vi "Test Convert.vi"(11 "Error in":errorcluster) -> (15 "Error out":errorcluster)   [LabVIEW 2020, in "CelsiusToFarenheitTests.lvlib"]
doc: "This VI is to validate Celsius to farenheit"
uses:
  CelsiusToFarenheitTests.lvlib
  <vilib>/addons/_JKI Toolkits/Caraya/classes/Test Suite/Define Test Suite (JUnit Report).vi
  <vilib>/SLL Drona/APIs/Stimulus/ControlValue/ValueSignalByPathString.vi
  <vilib>/SLL Drona/APIs/Assert/AssertControlValue/AlmostEqual.vi
  <vilib>/SLL Drona/APIs/Stimulus/VI/CloseVI.vi
  <vilib>/Utility/error.llb/Error Cluster From Error Code.vi
  <vilib>/ErrorRing/Error Ring.xnode
  <vilib>/addons/_JKI Toolkits/Caraya/classes/Test Suite/Test Suite.lvclass
  <vilib>/SLL Drona/Drona.lvlib
  <vilib>/addons/_JKI Toolkits/Caraya/classes/Test/Test.lvclass
  <vilib>/Wiresmith Technology/G CLI/CLI Class/CLI.lvclass
  <vilib>/SLL Drona/APIs/Assert/AssertControlValue/AssertControlValue.lvlib
  <vilib>/SLL Drona/APIs/Stimulus/ControlValue/ControlValue.lvlib
  <vilib>/SLL Drona/APIs/Stimulus/VI/VI.lvlib
panel:
  # "CELSIUS TO FARENHEIT TEST"
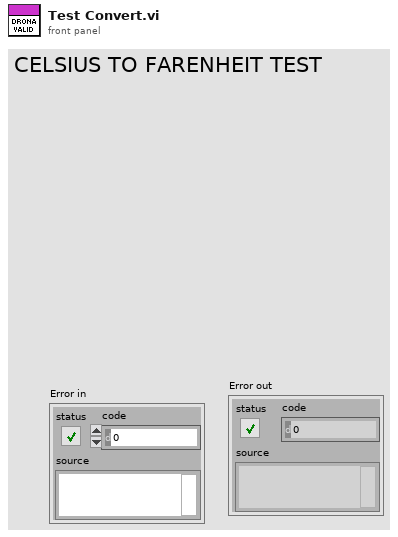
[diagram p1: front panel]
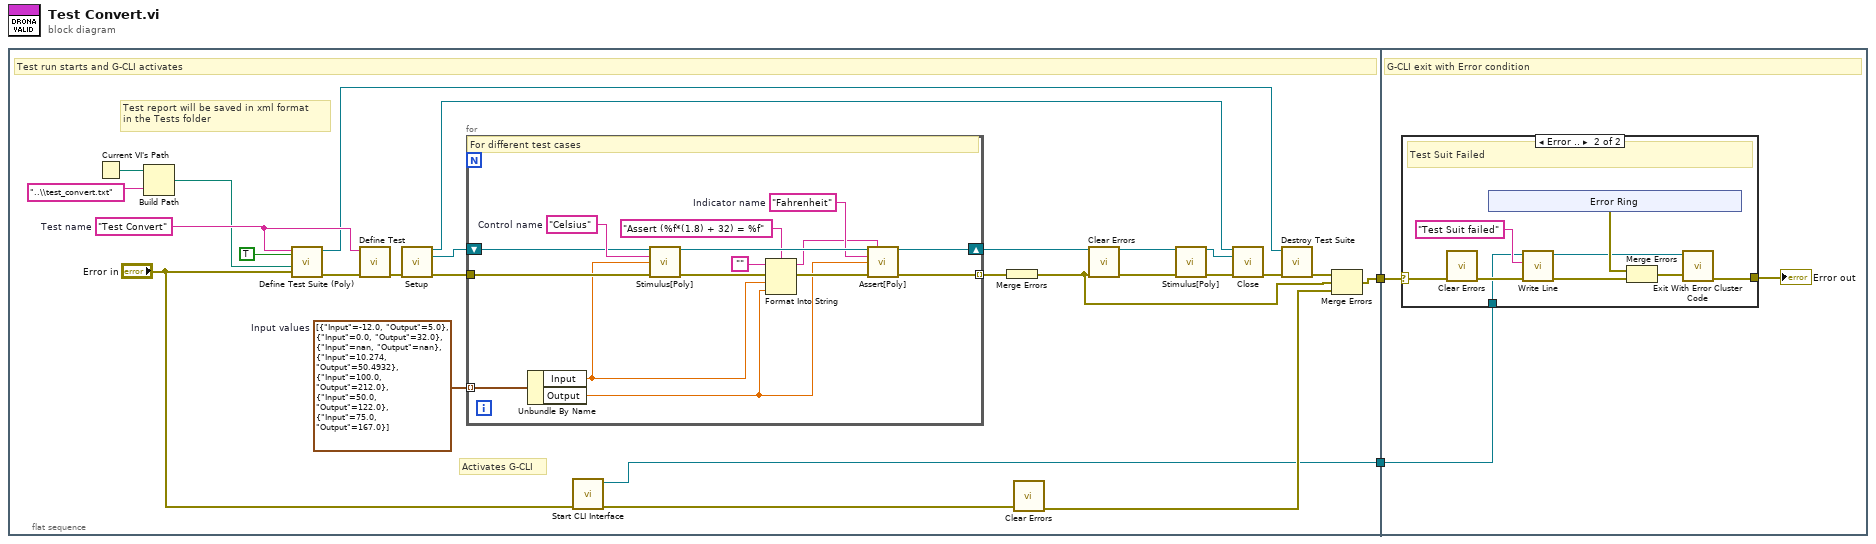
[diagram p0: block diagram]
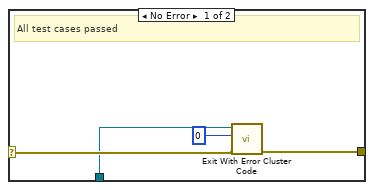
[diagram p2: hidden frame]
diagram:
  n1 = flat-sequence {
    tunnel: [w17] -> w2
    tunnel: [w15] -> w1
    tunnel: w2 -> [w45]
    tunnel: w1 -> [w43]
    frame #0 {
      w14 = "Test Convert"  # Test name
      w25 = cluster{"Input":dbl, "Output":dbl}[] [{"Input"=-12.0, "Output"=5.0}, {"Input"=0.0, "Output"=32.0}, {"Input"=nan, "Output"=nan}, {"Input"=10.274, "Output"=50.4932}, {"Input"=100.0, "Output"=212.0}, {"Input"=50.0, "Output"=122.0}, {"Input"=75.0, "Output"=167.0}]  # Input values
      # "Test report will be saved in xml format\nin the Tests folder"
      # "Activates G-CLI"
      # "Test run starts and G-CLI activates"
      n2 = Current VI's Path() -> (path=w10:path)
      n3 = Build Path(base path=w10, name or relative path="..\\test_convert.txt") -> (appended path=w8:path)
      n4 = call-poly <vilib>:"Define Test Suite (Poly).vi"("error in (no error)"="Error in", "Report Path"=w8, "Interactive"=TRUE, "Label (VI Title)"=w14) -> ("error out"=w13:errorcluster, "Test Suite"=w5:refnum<class "Test Suite.lvclass">)  [unwired: 6 in]
      n5 = call <vilib>:"Define Test.vi"("error in (no error)"=w13, "Label (VI Title)"=w14) -> ("error out"=w27:errorcluster)  [unwired: 9 in]
      n6 = call <vilib>:"Setup.vi"("error in"=w27) -> ("Application Ref"=w23:refnum<vi>, "VI Reference Out"=w24:refnum<vi>, "error out"=w26:errorcluster)  [unwired: 12 in]
      n7 = for {
        tunnel: w25 -> [w41] mode=indexing
        shift-right: [w31] -> w22
        shift-left: w24 -> [w39]
        tunnel: w26 -> [w42]
        tunnel: [w29] -> w19 mode=indexing
        w32 = "Fahrenheit"  # Indicator name
        w40 = "Celsius"  # Control name
        # "For different test cases"
        n8 = Unbundle By Name(w41) -> ("Input"=w28:dbl, "Output"=w33:dbl)
        n9 = call-poly <vilib>:"Stimulus[Poly].vi"("VI Reference In"=w39, "Control Path"=w40, "Value (Signaling)"=w28, "error in"=w42) -> ("VI Reference Out"=w35:refnum<vi>, "error out"=w37:errorcluster)  [unwired: 10 in]
        n10 = Format Into String(format string="Assert (%f*(1.8) + 32) = %f", initial string="", error in=w37, w28, w33) -> (resulting string=w30:string, error out=w36:errorcluster)
        n11 = call-poly <vilib>:"Assert[Poly].vi"("VI Reference In"=w35, "Test Label"=w30, "Control Path"=w32, "Control Value"=w33, "Error In"=w36) -> ("VI Reference Out"=w31:refnum<vi>, "Error Out"=w29:errorcluster)  [unwired: 9 in]
      }
      n12 = call <vilib>:"Start CLI Interface.vi"("error in (no error)"="Error in") -> ("error out"=w16:errorcluster, "CLI out"=w15:refnum<class "CLI.lvclass">)  [unwired: 7 in, 2 out]
      n13 = Merge Errors(w19) -> (w3:errorcluster)
      n14 = call <vilib>:"Clear Errors.vi"("error in (no error)"=w16) -> ("error out"=w18:errorcluster)  [unwired: 5 in, 1 out]
      n15 = call <vilib>:"Clear Errors.vi"("error in (no error)"=w3) -> ("error out"=w4:errorcluster)  [unwired: 5 in, 1 out]
      n16 = call-poly <vilib>:"Stimulus[Poly].vi"("VI Reference In"=w22, "error in"=w4) -> ("VI Reference Out"=w21:refnum<vi>, "error out"=w20:errorcluster)  [unwired: 12 in]
      n17 = call <vilib>:"Close.vi"("Application Ref"=w23, "VI Reference"=w21, "error in"=w20) -> ("error out"=w7:errorcluster)  [unwired: 12 in]
      n18 = call-dynamic "Destroy Test Suite.vi"("error in (no error)"=w7, "Test Suite in"=w5) -> ("error out"=w6:errorcluster)  [unwired: 8 in, 1 out]
      n19 = Merge Errors(w6, w3, w18) -> (w17:errorcluster)
    }
    frame #1 {
      # "G-CLI exit with Error condition"
      n20 = case shown="Error .." w45 {
        selector: w45 -> [w49 w56]
        tunnel: [w48 w58] -> w44
        tunnel: w43 -> [w46 w51]
        frame No Error {
          # "All test cases passed"
          n21 = call <vilib>:"Exit With Error Cluster Code.vi"("error in (no error)"=w49, "No Error Code (0)"=0, "CLI in"=w46) -> ("error out"=w48:errorcluster)  [unwired: 8 in]
        }
        frame Error {
          # "Test Suit Failed"
          n22 = call <vilib>:"Clear Errors.vi"("error in (no error)"=w56) -> ("error out"=w55:errorcluster)  [unwired: 5 in, 1 out]
          n23 = xnode "Error Ring"() -> ("error out"=w53:errorcluster)
          n24 = call <vilib>:"Write Line.vi"("error in (no error)"=w55, "Text to Write"="Test Suit failed", "CLI in"=w51) -> ("error out"=w52:errorcluster, "CLI out"=w50:refnum<class "CLI.lvclass">)  [unwired: 7 in]
          n25 = Merge Errors(w53, w52) -> (w54:errorcluster)
          n26 = call <vilib>:"Exit With Error Cluster Code.vi"("error in (no error)"=w54, "CLI in"=w50) -> ("error out"=w58:errorcluster)  [unwired: 9 in]
        }
      }
      "Error out" <- w44
    }
  }
